vi "Write TraceArray.vi"(8 "error in (no error)":errorcluster, 10 "TraceArray":T1(array[cluster]), 11 "SpecAnBase in":refnum<class "SpecAnBase.lvclass">) -> (0 "error out":errorcluster, 3 "SpecAnBase out":refnum<class "SpecAnBase.lvclass">)   [LabVIEW 2014]
uses:
  SpecAnBase.lvclass
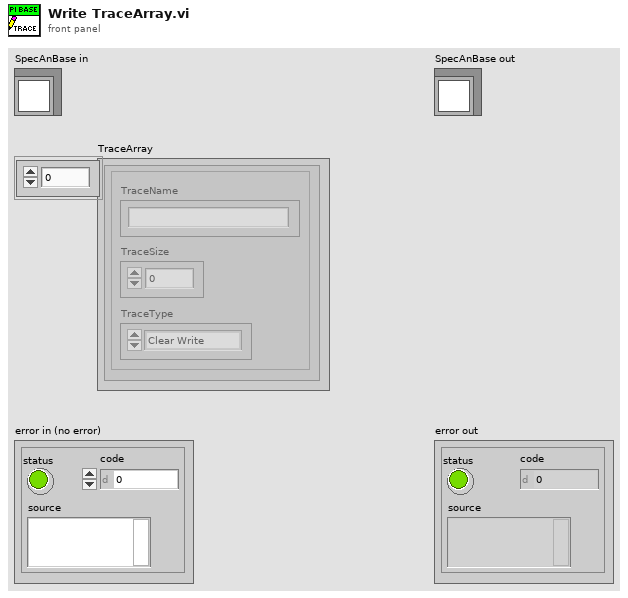
[diagram p1: front panel]
types:
  T1 = cluster{"TraceName":string, "TraceSize":i32, "TraceType":enum16{"Clear Write", "Maximum Hold", "Minimum Hold", "Video Average", "View", "Store"}}[]
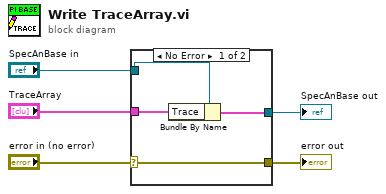
[diagram p0: block diagram]
diagram:
  n1 = case shown="No Error" "error in (no error)" {
    selector: "error in (no error)" -> [w9 w10]
    tunnel: [w9 w10] -> w4
    tunnel: [w7 w11] -> w2
    tunnel: "SpecAnBase in" -> [w8 w11]
    tunnel: "TraceArray" -> [w6 _]
    frame No Error {
      n2 = Bundle By Name(cluster=w8, "Trace"=w6) -> (w7:cluster{})
    }
    frame Error {
    }
  }
  "error out" <- w4
  "SpecAnBase out" <- w2
